vi "DIO Configure.vi"(8 "error in (no error)":errorcluster, 10 "Params":variant, 11 "NI Digital IO in":refnum<class "NI Digital IO.lvclass">) -> (0 "error out":errorcluster, 3 "NI Digital IO out":refnum<class "NI Digital IO.lvclass">)   [LabVIEW 2020, in "NI DAQmx.lvlib" / "NI Digital IO.lvclass"]
uses:
  NI Digital IO.lvclass
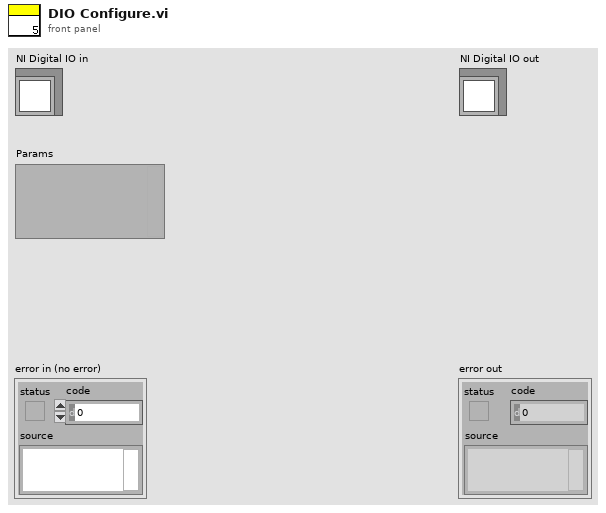
[diagram p1: front panel]
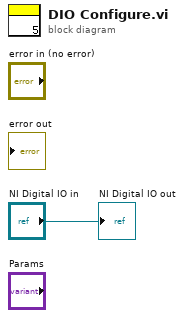
[diagram p0: block diagram]
diagram:
  "NI Digital IO out" <- "NI Digital IO in"
